vi "Configure Measurement.vi"(6 "Manual Range (1.0)":dbl=1.0, 7 "Manual Resolution (5.5 Digits)":dbl(ring)=5.5 items=["4.5"=4.5, "5.5"=5.5, "6.5"=6.5], 8 "error in (no error)":errorcluster, 9 "Auto Range (T:Enable)":bool=TRUE, 10 "Function (0: DC Voltage)":u16(ring) items=["DC Voltage", "AC Voltage", "2 - Wire Resistance", "4 - Wire Resistance", "DC Current", "AC Current", "Frequency", "Period", "Continuity", "Diode Checking", "Temperature", "Capacitance"], 11 "VISA resource name":refnum<visa-resource-name>) -> (0 "error out":errorcluster, 3 "VISA resource name out":refnum<visa-resource-name>)   [LabVIEW 2014, in "Fluke 884X Series.lvlib"]
doc: "Configures the measurement type, resolution, and range on the instrument.\n\n<B>Note:</B>\n\nFluke 8845A does not support Temperature or Capacitance configurations or measurements."
uses:
  Fluke 884X Series.lvlib
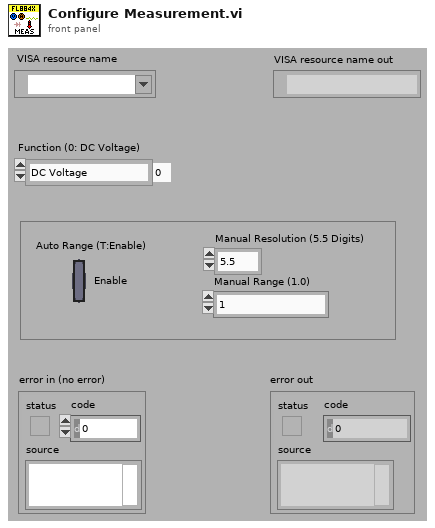
[diagram p1: front panel]
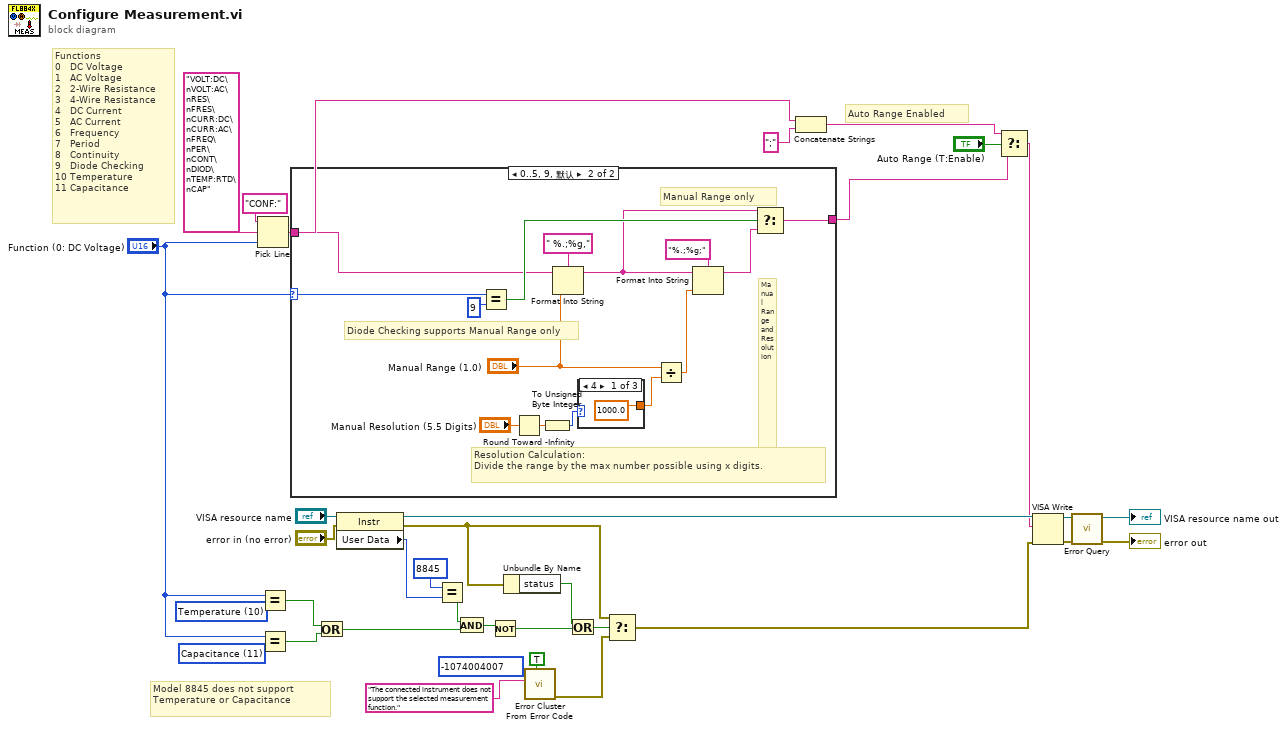
[diagram p0: block diagram]
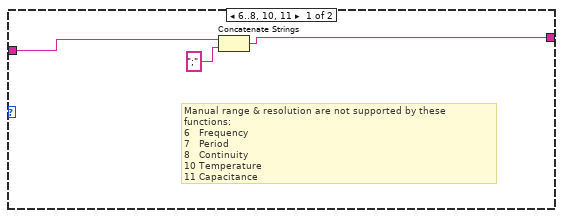
[diagram p2: hidden frame]
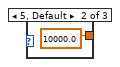
[diagram p3: hidden frame]
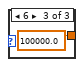
[diagram p4: hidden frame]
diagram:
  w12 = u16 11 items=["DC Voltage", "AC Voltage", "2 - Wire Resistance", "4 - Wire Resistance", "DC Current", "AC Current", "Frequency", "Period", "Continuity", "Diode Checking", "Temperature", "Capacitance"] ("Function (0: DC Voltage)")
  w14 = u16 10 items=["DC Voltage", "AC Voltage", "2 - Wire Resistance", "4 - Wire Resistance", "DC Current", "AC Current", "Frequency", "Period", "Continuity", "Diode Checking", "Temperature", "Capacitance"] ("Function (0: DC Voltage)")
  # "Model 8845 does not support\nTemperature or Capacitance"
  # "Auto Range Enabled"
  # "Functions\n0   DC Voltage   \n1   AC Voltage                            \n2   2-Wire Resistance          \n3   4-Wire Resistance         \n4   DC Current        \n5   AC Current\n6   Frequency\n7   Period          \n8   Continuity\n9   Diode Checking \n10 Temperature \n11 Capacitance"
  n1 = Pick Line(string ("")="CONF:", multi-line string="VOLT:DC\nVOLT:AC\nRES\nFRES\nCURR:DC\nCURR:AC\nFREQ\nPER\nCONT\nDIOD\nTEMP:RTD\nCAP", line index="Function (0: DC Voltage)") -> (output string=w23:string)
  n2 = Equal?(x="Function (0: DC Voltage)", y=w14) -> (x = y?=w13:bool)
  n3 = Equal?(x="Function (0: DC Voltage)", y=w12) -> (x = y?=w10:bool)
  n4 = case shown="0..5, 9, 默认" "Function (0: DC Voltage)" {
    selector: "Function (0: DC Voltage)" -> [_ w45]
    tunnel: w23 -> [w36 w44]
    tunnel: [w35 w43] -> w24
    frame 6..8, 10, 11 {
      # "Manual range & resolution are not supported by these functions:\n6   Frequency\n7   Period\n8   Continuity\n10 Temperature\n11 Capacitance"
      n5 = Concatenate Strings(w36, ";" ("string")) -> (w35:string)
    }
    frame 0..5, 9, Default {
      # "Manual Range only"
      # "Resolution Calculation: \nDivide the range by the max number possible using x digits."
      # "Diode Checking supports Manual Range only"
      # "Manual Range and Resolution"
      n6 = Equal?(x=w45, y=9) -> (x = y?=w46:bool)
      n7 = Round Toward -Infinity(1:"Manual Resolution (5.5 Digits)") -> (0:w41:dbl)
      n8 = To Unsigned Byte Integer(number=w41) -> (unsigned 8bit integer=w52:u8)
      n9 = Format Into String(format string=" %.;%g,", initial string=w44, "Manual Range (1.0)") -> (resulting string=w38:string)  [unwired: 1 in, 1 out]
      n10 = case shown="4" w52 {
        tunnel: [1000.0 10000.0 100000.0] -> w50
        frame 4 {
        }
        frame 5, Default {
        }
        frame 6 {
        }
      }
      n11 = Divide(x="Manual Range (1.0)", y=w50) -> (x/y=w51:dbl)
      n12 = Format Into String(format string="%.;%g;", initial string=w38, w51) -> (resulting string=w48:string)  [unwired: 1 in, 1 out]
      n13 = Select(t=w38, s=w46, f=w48) -> (s? t:f=w43:string)
    }
  }
  n14 = Or(x=w13, y=w10) -> (x .or. y?=w9:bool)
  n15 = property class="Instr"(reference="VISA resource name", error in="error in (no error)") -> (reference out=w16:refnum<visa-resource-name>, error out=w3:errorcluster, "User Data"=w17:u32)
  n16 = Equal?(x=u32 8845, y=w17) -> (x = y?=w15:bool)
  n17 = And(x=w15, y=w9) -> (x .and. y?=w7:bool)
  n18 = Not(x=w7) -> (.not. x?=w5:bool)
  n19 = Unbundle By Name(w3) -> ("status"=w6:bool)
  n20 = call <vilib>:"Error Cluster From Error Code.vi"("show call chain? (False)"=TRUE, "error message (\"\")"="The connected instrument does not support the selected measurement function." ("Source (VI Name)"), "error code (0)"=-1074004007 ("Code")) -> ("error out"=w2:errorcluster)  [unwired: 6 in]
  n21 = Or(x=w6, y=w5) -> (x .or. y?=w4:bool)
  n22 = Select(t=w3, s=w4, f=w2) -> (s? t:f=w1:errorcluster)
  n23 = Concatenate Strings(w23, ";" ("string")) -> (w26:string)
  n24 = Select(t=w26, s="Auto Range (T:Enable)", f=w24) -> (s? t:f=w8:string)
  n25 = VISA Write(VISA resource name=w16, write buffer=w8, error in (no error)=w1) -> (VISA resource name out=w32:refnum<visa-resource-name>, error out=w31:errorcluster)  [unwired: 1 out]
  n26 = call "Error Query.vi"("error in (no error)"=w31, "VISA resource name"=w32) -> ("error out"=→"error out":errorcluster, "VISA resource name out"=→"VISA resource name out":refnum<visa-resource-name>)  [unwired: 6 in, 2 out]
